vi "Slew Rate.vi"(8 "错误输入（无错误）":errorcluster, 11 "Analog Waveforms":waveform(dbl)[](array[waveform])) -> (0 "错误输出":errorcluster, 2 "Dynamic Data":dynamicdata(waveform), 3 "waveform":waveform(dbl))   [LabVIEW 2019]
uses:
  <vilib>/Waveform/WDTOps.llb/WDT Index Channel DBL.vi
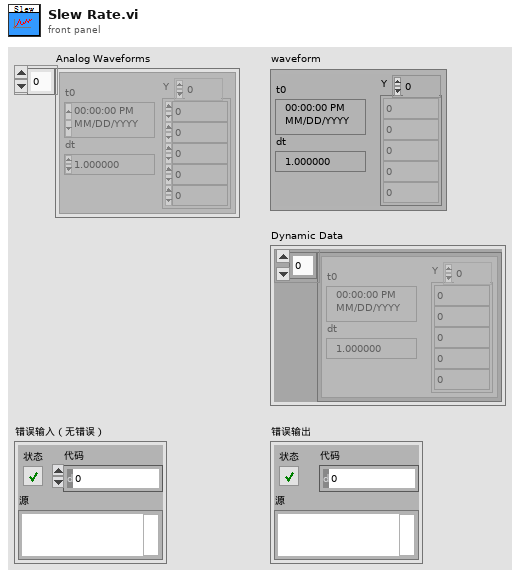
[diagram p1: front panel]
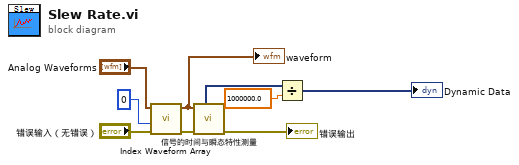
[diagram p0: block diagram]
diagram:
  n1 = call-poly <vilib>:"Index Waveform Array.vi"("error in (no error)"="错误输入（无错误）", "index"=0, "waveform array"="Analog Waveforms") -> ("error out"=w8:errorcluster, "waveform"=w7:waveform(dbl))  [unwired: 7 in]
  "waveform" <- w7
  n2 = call "信号的时间与瞬态特性测量"("error in (no error)"=w8, "Signals"=w7) -> ("error out"=→"错误输出":errorcluster, "Slew Rate"=w4:dynamicdata)  [unwired: 8 in]
  n3 = Divide(x=w4, y=1000000.0) -> (x/y=→"Dynamic Data":dynamicdata)
